vi "util_get_config_path.vi"(8 "error in (no error)":errorcluster) -> (0 "error out":errorcluster, 3 "lv_build_config_path":path)   [LabVIEW 2015, in "lv-build.lvlib"]
uses:
  <vilib>/Utility/sysdir.llb/System Directory Type.ctl
  lv-build.lvlib
  <userlib>/antonio-alexander/lv-bin/public/api/v1/v1.lvlib
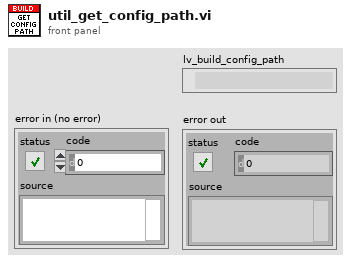
[diagram p1: front panel]
types:
  T1 = typedef "System Directory Type.ctl" = i32
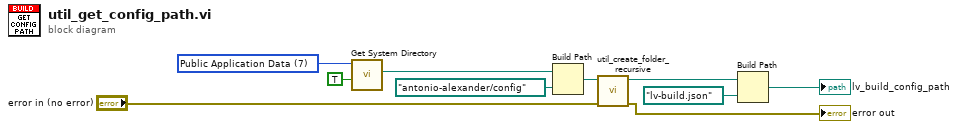
[diagram p0: block diagram]
diagram:
  w10 = T1 7 items=["User Home"=0, "User Desktop"=1, "User Documents"=2, "User Application Data"=3, "User Preferences"=4, "User Temporary"=5, "Public Documents"=6, "Public Application Data"=7, "Public Preferences"=8, "Public Cache"=13, "System Core Libraries"=9, "System Installed Libraries"=10, "Application Files"=11, "Boot Volume Root"=12] ("system directory type")
  n1 = call <vilib>:"Get System Directory.vi"("create directory if not found? (F)"=TRUE, "system directory type"=w10) -> ("system directory"=w8:path)  [unwired: 9 in]
  n2 = Build Path(base path=w8, name or relative path=path "antonio-alexander/config" ("system directory")) -> (appended path=w6:path)
  n3 = call <userlib>:"util_create_folder_recursive.vi"("error in"="error in (no error)", "path in"=w6) -> ("error out"=→"error out":errorcluster, "path out"=w5:path)  [unwired: 8 in]
  n4 = Build Path(base path=w5, name or relative path=path "lv-build.json" ("system directory")) -> (appended path=→"lv_build_config_path":path)
